vi "GetPosition.vi"(3 "error in":errorcluster, 5 "VISA resource name in":refnum<visa-resource-name>) -> (0 "error out":errorcluster, 1 "Position XYZ":dbl[](array[numeric]), 2 "VISA resource name out":refnum<visa-resource-name>)   [LabVIEW 2016]
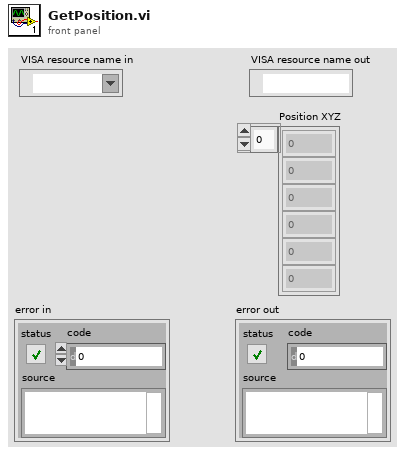
[diagram p1: front panel]
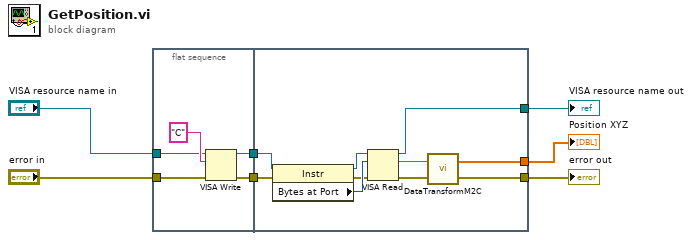
[diagram p0: block diagram]
diagram:
  n1 = flat-sequence {
    tunnel: [w11] -> w7
    tunnel: [w10] -> w6
    tunnel: "VISA resource name in" -> [w9]
    tunnel: "error in" -> [w8]
    tunnel: w7 -> [w20]
    tunnel: [w19] -> w2
    tunnel: w6 -> [w18]
    tunnel: [w14] -> w1
    tunnel: [w13] -> w3
    frame #0 {
      n2 = VISA Write(VISA resource name=w9, write buffer="C", error in (no error)=w8) -> (VISA resource name out=w11:refnum<visa-resource-name>, error out=w10:errorcluster)  [unwired: 1 out]
    }
    frame #1 {
      n3 = property class="Instr"(reference=w20, error in=w18) -> (reference out=w22:refnum<visa-resource-name>, error out=w17:errorcluster, "Bytes at Port"=w21:u32)
      n4 = VISA Read(VISA resource name=w22, byte count=w21, error in (no error)=w17) -> (VISA resource name out=w19:refnum<visa-resource-name>, read buffer=w16:string, error out=w15:errorcluster)  [unwired: 1 out]
      n5 = call "DataTransformM2C.vi"("ERROR IN"=w15, "MotorData"=w16) -> ("ERROR OUT"=w14:errorcluster, "Computer Data"=w13:dbl[])
    }
  }
  "Position XYZ" <- w3
  "VISA resource name out" <- w2
  "error out" <- w1
